vi "imaqrio_RunMethImpl.vi"(3 "error in (no error)":errorcluster, 4 "reference":refnum<visa-resource-name>) -> (0 "error out":errorcluster, 1 "dup reference":refnum<visa-resource-name>)   [LabVIEW 2017]
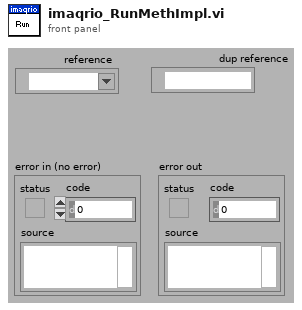
[diagram p1: front panel]
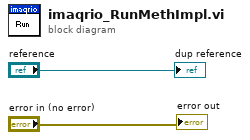
[diagram p0: block diagram]
diagram:
  "error out" <- "error in (no error)"
  "dup reference" <- "reference"
